vi "Zoom_graph (SubVI).vi"(9 "Delta":i32, 10 "Param":cluster{"max":dbl, "increment":dbl}={"max"=1.4, "increment"=0.025}, 11 "YScale.Range in":T1) -> (2 "Boolean":bool, 3 "YScale.Range out":T1)   [LabVIEW 2017]
uses:
  <vilib>/Utility/miscctls.llb/LVRangeTypeDef.ctl
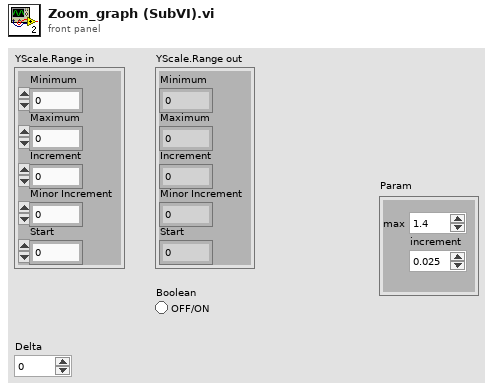
[diagram p1: front panel]
types:
  T1 = typedef "LVRangeTypeDef.ctl" = cluster{"Minimum":dbl, "Maximum":dbl, "Increment":dbl, "Minor Increment":dbl, "Start":dbl}
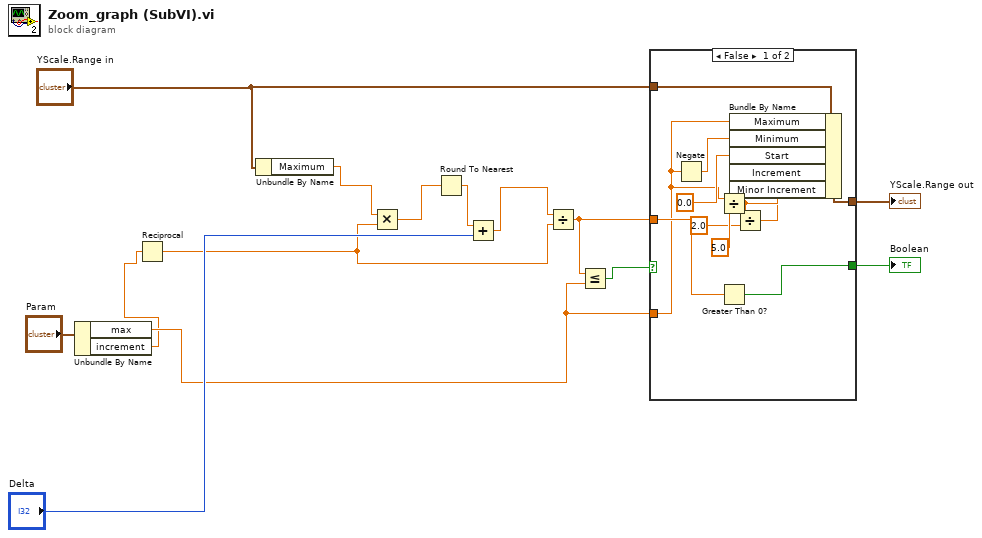
[diagram p0: block diagram]
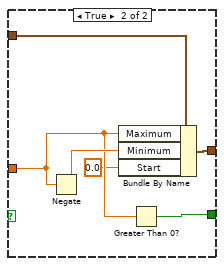
[diagram p2: hidden frame]
diagram:
  n1 = Unbundle By Name("Param") -> ("max"=w2:dbl, "increment"=w1:dbl)
  n2 = Reciprocal(x=w1) -> (1/x=w6:dbl)
  n3 = Unbundle By Name("YScale.Range in") -> ("Maximum"=w7:dbl)
  n4 = Multiply(x=w7, y=w6) -> (x*y=w8:dbl)
  n5 = Round To Nearest(number=w8) -> (nearest integer value=w9:dbl)
  n6 = Add(x=w9, y="Delta") -> (x+y=w10:dbl)
  n7 = Divide(x=w10, y=w6) -> (x/y=w5:dbl)
  n8 = Less Or Equal?(x=w5, y=w2) -> (x <= y?=w4:bool)
  n9 = case shown="False" w4 {
    tunnel: [w24 w31] -> w14
    tunnel: [w22 w30] -> w13
    tunnel: "YScale.Range in" -> [w23 w28]
    tunnel: w5 -> [w25 w27]
    tunnel: w2 -> [w19 _]
    frame False {
      n10 = Negate(x=w19) -> (-x=w21:dbl)
      n11 = Divide(x=w19, y=5.0) -> (x/y=w17:dbl)
      n12 = Greater Than 0?(x=w25) -> (x > 0?=w24:bool)
      n13 = Divide(x=w17, y=2.0) -> (x/y=w15:dbl)
      n14 = Bundle By Name(cluster=w23, "Maximum"=w19, "Minimum"=w21, "Start"=0.0, "Increment"=w17, "Minor Increment"=w15) -> (w22:T1)
    }
    frame True {
      n15 = Negate(x=w27) -> (-x=w29:dbl)
      n16 = Bundle By Name(cluster=w28, "Maximum"=w27, "Minimum"=w29, "Start"=0.0) -> (w30:T1)
      n17 = Greater Than 0?(x=w27) -> (x > 0?=w31:bool)
    }
  }
  "Boolean" <- w14
  "YScale.Range out" <- w13
